vi "Get_Item.MCListboxArray.vi"(7 "SelctionType":i32[](array[numeric]), 8 "error in (no error)":errorcluster, 10 "Control Label":string, 11 "Data Value Reference in":T1) -> (0 "error out":errorcluster, 2 "Items":string[][](array[string]), 3 "Data Value Reference out":T1)   [LabVIEW 2020, in "CtlReferences.lvlib" / "CtlReferences.lvclass"]
uses:
  CtlReferences.lvclass
  TypeDefs/CtlLookup.ctl
  GetControlRef/GetControl_MultiColumnListBox.vi
  GetCtlRef.vi
  Error_CtlNotFound.vi
  <vilib>/Utility/error.llb/Error Cluster From Error Code.vi
  Error_ToSpecificClass.vi
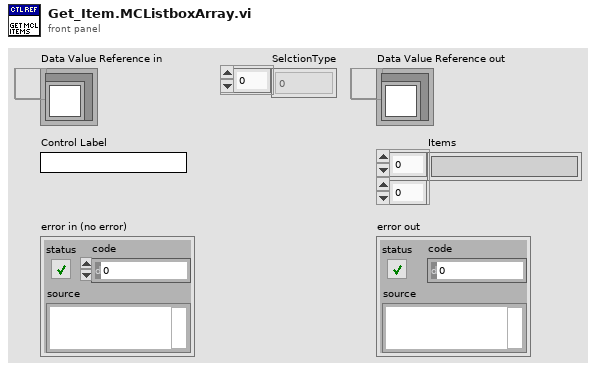
[diagram p1: front panel]
types:
  T1 = typedef "CtlReferences.lvlib/CtlReferences.lvclass/CtlLookup.ctl" = refnum<data-value>
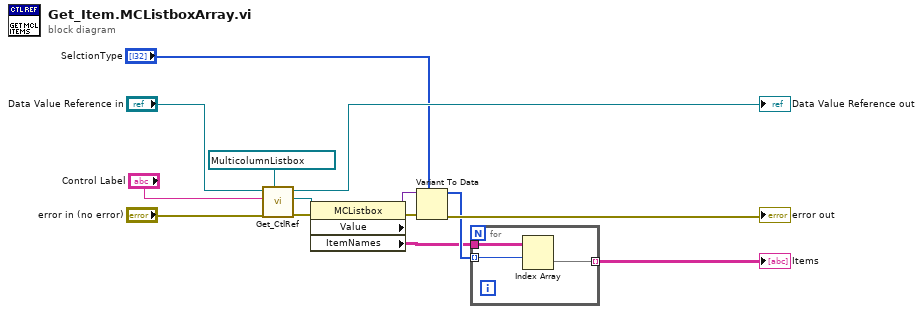
[diagram p0: block diagram]
diagram:
  n1 = call-poly "Get_CtlRef.vi"("Control Class"=refnum<vi> refnum, "error in (no error)"="error in (no error)", "Control Label"="Control Label", "CtlLookup In"="Data Value Reference in") -> ("error out"=w4:errorcluster, "Reference Out"=w5:refnum<vi>, "CtlLookup Out"=→"Data Value Reference out":T1)  [unwired: 5 in]
  n2 = property class="MCListbox"(reference=w5, error in=w4) -> (error out=w6:errorcluster, "Value"=w7:variant, "ItemNames"=w9:string[][])  [unwired: 1 out]
  n3 = Variant To Data(error in=w6, type="SelctionType", Variant=w7) -> (data=w10:i32[], error out=→"error out":errorcluster)
  n4 = for {
    tunnel: [w17] -> w12 mode=indexing
    tunnel: w10 -> [w16] mode=indexing
    tunnel: w9 -> [w15]
    n5 = Index Array(array=w15, index (row)=w16) -> (element=w17:string[])  [unwired: 1 in]
  }
  "Items" <- w12
